vi "机械臂参数配置（数组）.vi"() -> (0 "机械臂臂长":dbl[](array[numeric]), 1 "转轴最大角度":dbl[](array[numeric]), 2 "转轴最小角度":dbl[](array[numeric]))   [LabVIEW 2014]
uses:
  <vilib>/Utility/file.llb/Write To Spreadsheet File (DBL).vi
  <vilib>/Utility/file.llb/Read From Spreadsheet File (DBL).vi
panel:
  in  "取消按钮":bool
  in  "打开配置":bool
  in  "保存配置":bool
  in  "确定":bool
  out "读取机械臂臂长":dbl[](array[numeric])
  out "读取最大角度":dbl[](array[numeric])
  out "读取轴最小角度":dbl[](array[numeric])
  out "读取数据":dbl[][](array[numeric]) caption="所有行" format="%0.3f"
  out "数据":dbl[][](array[numeric])
  out "机械臂臂长2":dbl[](array[numeric])
  out "转轴最大角度2":dbl[](array[numeric])
  out "转轴最小角度2":dbl[](array[numeric])
  in  "Arm-4":dbl
  in  "Arm-3":dbl
  in  "Arm-2":dbl
  in  "Arm-1":dbl
  in  "3-Axi max":dbl
  in  "3-Axi min":dbl
  in  "2-Axi max":dbl
  in  "2-Axi min":dbl
  in  "6-Axi max":dbl
  in  "6-Axi min":dbl
  in  "5-Axi max":dbl
  in  "5-Axi min":dbl
  in  "4-Axi max":dbl
  in  "4-Axi min":dbl
  in  "1-Axi max":dbl
  in  "1-Axi min":dbl
  # "机器臂参数设置"
  # "机械臂臂长（mm）："
  # "机械臂-4"
  # "机械臂-3"
  # "机械臂-2"
  # "机械臂-1"
  # "最大角度（°）："
  # "最小角度（°）："
  # "转轴-3"
  # "转轴-2"
  # "转轴-6"
  # "转轴-5"
  # "转轴-4"
  # "转轴-1"
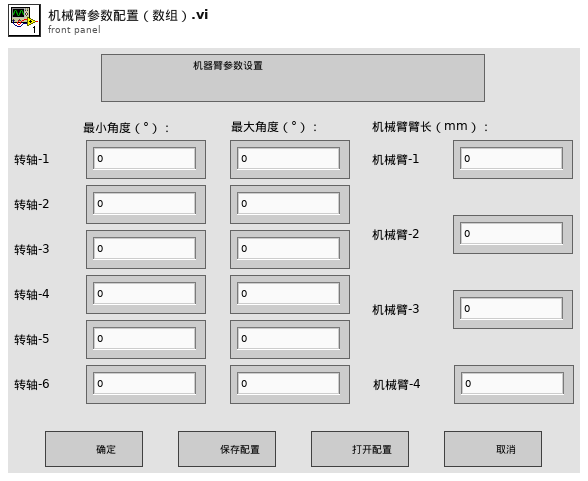
[diagram p1: front panel]
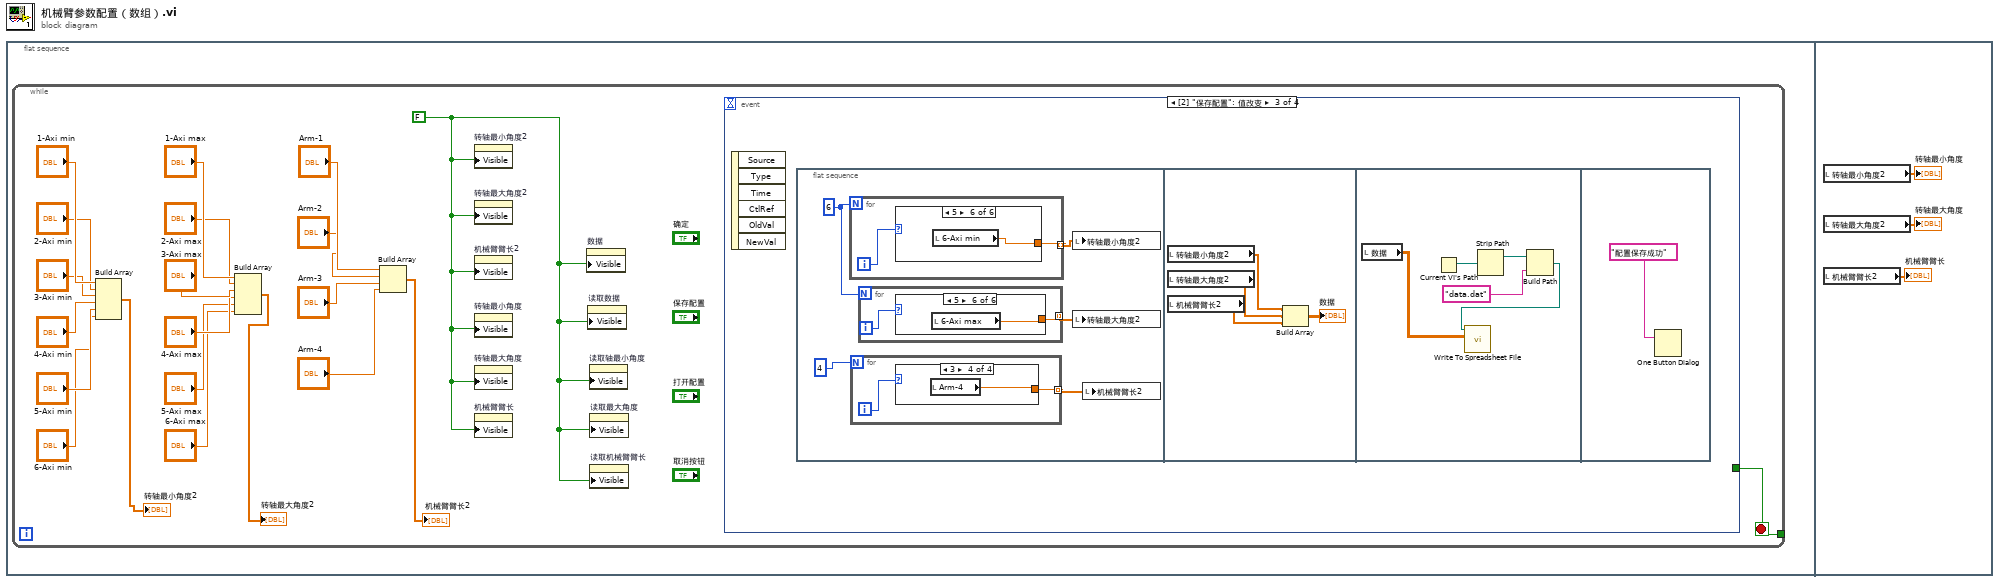
[diagram p0: block diagram]
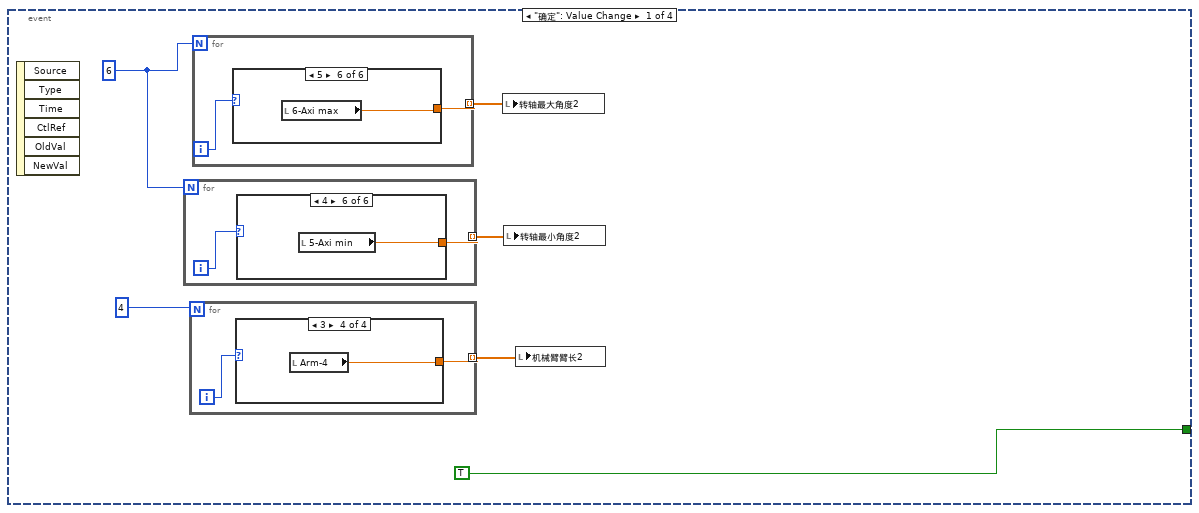
[diagram p2: hidden frame]
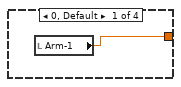
[diagram p3: hidden frame]
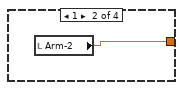
[diagram p4: hidden frame]
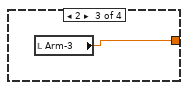
[diagram p5: hidden frame]
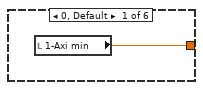
[diagram p6: hidden frame]
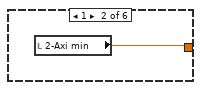
[diagram p7: hidden frame]
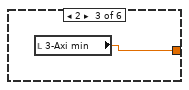
[diagram p8: hidden frame]
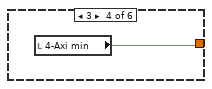
[diagram p9: hidden frame]
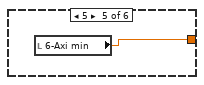
[diagram p10: hidden frame]
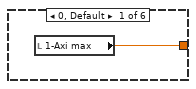
[diagram p11: hidden frame]
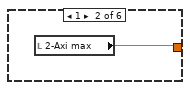
[diagram p12: hidden frame]
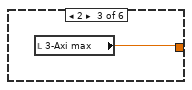
[diagram p13: hidden frame]
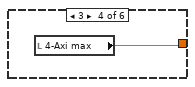
[diagram p14: hidden frame]
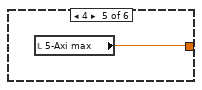
[diagram p15: hidden frame]
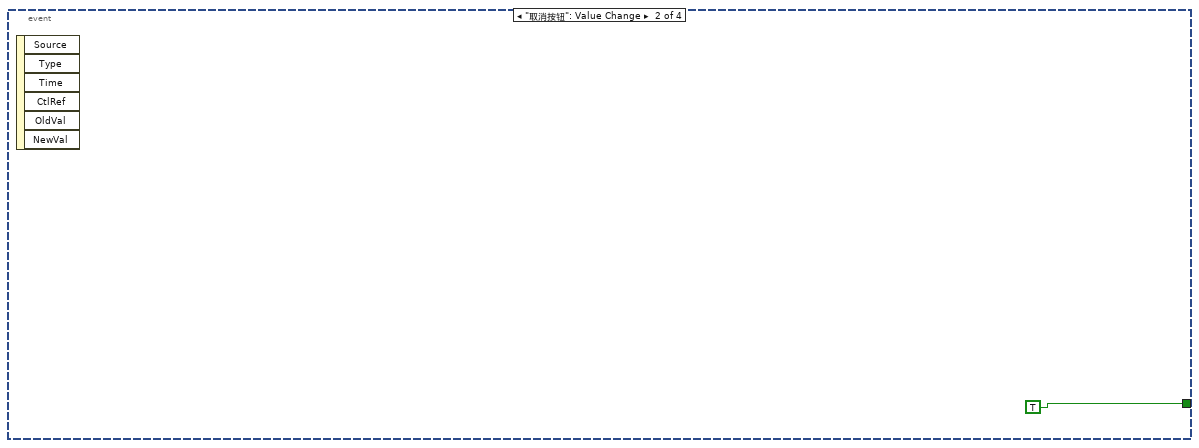
[diagram p16: hidden frame]
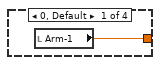
[diagram p17: hidden frame]
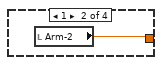
[diagram p18: hidden frame]
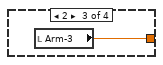
[diagram p19: hidden frame]
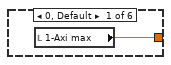
[diagram p20: hidden frame]
diagram:
  n1 = flat-sequence {
    frame #0 {
      n2 = while {
        tunnel: [w5] -> _
        stop <- w5 stop-if-true
        w4 = FALSE
        n3 = Build Array("1-Axi min", "2-Axi min", "3-Axi min", "4-Axi min", "5-Axi min", "6-Axi min") -> (→"转轴最小角度2":dbl[])
        n4 = Build Array("1-Axi max", "2-Axi max", "3-Axi max", "4-Axi max", "5-Axi max", "6-Axi max") -> (→"转轴最大角度2":dbl[])
        n5 = Build Array("Arm-1", "Arm-2", "Arm-3", "Arm-4") -> (→"机械臂臂长2":dbl[])
        n6 = property on="转轴最小角度2" class="Arr (严格)"("Visible"=w4) -> ()  [unwired: 2 in, 2 out]
        n7 = property on="转轴最大角度2" class="Arr (严格)"("Visible"=w4) -> ()  [unwired: 2 in, 2 out]
        n8 = property on="机械臂臂长2" class="Arr (严格)"("Visible"=w4) -> ()  [unwired: 2 in, 2 out]
        n9 = property on="转轴最小角度" class="Arr (严格)"("Visible"=w4) -> ()  [unwired: 2 in, 2 out]
        n10 = property on="转轴最大角度" class="Arr (严格)"("Visible"=w4) -> ()  [unwired: 2 in, 2 out]
        n11 = property on="机械臂臂长" class="Arr (严格)"("Visible"=w4) -> ()  [unwired: 2 in, 2 out]
        n12 = property on="数据" class="Arr (严格)"("Visible"=w4) -> ()  [unwired: 2 in, 2 out]
        n13 = property on="读取数据" class="Arr (严格)"("Visible"=w4) -> ()  [unwired: 2 in, 2 out]
        n14 = property on="读取轴最小角度" class="Arr (严格)"("Visible"=w4) -> ()  [unwired: 2 in, 2 out]
        n15 = property on="读取最大角度" class="Arr (严格)"("Visible"=w4) -> ()  [unwired: 2 in, 2 out]
        n16 = property on="读取机械臂臂长" class="Arr (严格)"("Visible"=w4) -> ()  [unwired: 2 in, 2 out]
        n17 = event shown="[2] \"保存配置\": 值改变" {
          selector: _ -> [_ _ _ _]
          dyn-events: _ -> [_ _ _ _]
          timeout: _ -> [_ _ _ _]
          tunnel: [TRUE TRUE _ _] -> w5
          event "确定": Value Change {
            w25 = 6
            n18 = event-data() -> ()  [unwired: 1 in, 6 out]
            n19 = for {
              N: w25 -> [_]
              tunnel: [w34] -> w24 mode=indexing
              i -> [w35]
              n20 = case shown="4" w35 {
                tunnel: [w36 w37 w38 w39 w40 w41] -> w34
                frame 0, Default {
                  n21 = local read "1-Axi min"() -> (w36:dbl)
                }
                frame 1 {
                  n22 = local read "2-Axi min"() -> (w37:dbl)
                }
                frame 2 {
                  n23 = local read "3-Axi min"() -> (w38:dbl)
                }
                frame 3 {
                  n24 = local read "4-Axi min"() -> (w39:dbl)
                }
                frame 5 {
                  n25 = local read "6-Axi min"() -> (w40:dbl)
                }
                frame 4 {
                  n26 = local read "5-Axi min"() -> (w41:dbl)
                }
              }
            }
            n27 = for {
              N: 4 -> [_]
              tunnel: [w28] -> w22 mode=indexing
              i -> [w29]
              n28 = case shown="3" w29 {
                tunnel: [w30 w31 w32 w33] -> w28
                frame 0, Default {
                  n29 = local read "Arm-1"() -> (w30:dbl)
                }
                frame 1 {
                  n30 = local read "Arm-2"() -> (w31:dbl)
                }
                frame 2 {
                  n31 = local read "Arm-3"() -> (w32:dbl)
                }
                frame 3 {
                  n32 = local read "Arm-4"() -> (w33:dbl)
                }
              }
            }
            n33 = for {
              N: w25 -> [_]
              tunnel: [w42] -> w26 mode=indexing
              i -> [w43]
              n34 = case shown="5" w43 {
                tunnel: [w44 w45 w46 w47 w48 w49] -> w42
                frame 0, Default {
                  n35 = local read "1-Axi max"() -> (w44:dbl)
                }
                frame 1 {
                  n36 = local read "2-Axi max"() -> (w45:dbl)
                }
                frame 2 {
                  n37 = local read "3-Axi max"() -> (w46:dbl)
                }
                frame 3 {
                  n38 = local read "4-Axi max"() -> (w47:dbl)
                }
                frame 4 {
                  n39 = local read "5-Axi max"() -> (w48:dbl)
                }
                frame 5 {
                  n40 = local read "6-Axi max"() -> (w49:dbl)
                }
              }
            }
            n41 = local write "转轴最大角度2"(w26) -> ()
            n42 = local write "转轴最小角度2"(w24) -> ()
            n43 = local write "机械臂臂长2"(w22) -> ()
          }
          event "取消按钮": Value Change {
            n44 = event-data() -> ()  [unwired: 1 in, 6 out]
          }
          event "保存配置": Value Change {
            n45 = event-data() -> ()  [unwired: 1 in, 6 out]
            n46 = flat-sequence {
              frame #0 {
                w55 = 6
                n47 = for {
                  N: w55 -> [_]
                  tunnel: [w70] -> w53 mode=indexing
                  i -> [w71]
                  n48 = case shown="5" w71 {
                    tunnel: [w72 w73 w74 w75 w76 w77] -> w70
                    frame 0, Default {
                      n49 = local read "1-Axi min"() -> (w72:dbl)
                    }
                    frame 1 {
                      n50 = local read "2-Axi min"() -> (w73:dbl)
                    }
                    frame 2 {
                      n51 = local read "3-Axi min"() -> (w74:dbl)
                    }
                    frame 3 {
                      n52 = local read "4-Axi min"() -> (w75:dbl)
                    }
                    frame 4 {
                      n53 = local read "5-Axi min"() -> (w76:dbl)
                    }
                    frame 5 {
                      n54 = local read "6-Axi min"() -> (w77:dbl)
                    }
                  }
                }
                n55 = for {
                  N: 4 -> [_]
                  tunnel: [w56] -> w51 mode=indexing
                  i -> [w57]
                  n56 = case shown="3" w57 {
                    tunnel: [w58 w59 w60 w61] -> w56
                    frame 0, Default {
                      n57 = local read "Arm-1"() -> (w58:dbl)
                    }
                    frame 1 {
                      n58 = local read "Arm-2"() -> (w59:dbl)
                    }
                    frame 2 {
                      n59 = local read "Arm-3"() -> (w60:dbl)
                    }
                    frame 3 {
                      n60 = local read "Arm-4"() -> (w61:dbl)
                    }
                  }
                }
                n61 = for {
                  N: w55 -> [_]
                  tunnel: [w62] -> w52 mode=indexing
                  i -> [w63]
                  n62 = case shown="5" w63 {
                    tunnel: [w64 w65 w66 w67 w68 w69] -> w62
                    frame 0, Default {
                      n63 = local read "1-Axi max"() -> (w64:dbl)
                    }
                    frame 1 {
                      n64 = local read "2-Axi max"() -> (w65:dbl)
                    }
                    frame 2 {
                      n65 = local read "3-Axi max"() -> (w66:dbl)
                    }
                    frame 3 {
                      n66 = local read "4-Axi max"() -> (w67:dbl)
                    }
                    frame 4 {
                      n67 = local read "5-Axi max"() -> (w68:dbl)
                    }
                    frame 5 {
                      n68 = local read "6-Axi max"() -> (w69:dbl)
                    }
                  }
                }
                n69 = local write "转轴最小角度2"(w53) -> ()
                n70 = local write "转轴最大角度2"(w52) -> ()
                n71 = local write "机械臂臂长2"(w51) -> ()
              }
              frame #1 {
                n72 = local read "转轴最小角度2"() -> (w81:dbl[])
                n73 = local read "转轴最大角度2"() -> (w80:dbl[])
                n74 = local read "机械臂臂长2"() -> (w79:dbl[])
                n75 = Build Array(w81, w80, w79) -> (→"数据":dbl[][])
              }
              frame #2 {
                n76 = local read "数据"() -> (w86:dbl[][])
                n77 = Current VI's Path() -> (path=w85:path)
                n78 = Strip Path(path=w85) -> (stripped path=w84:path)  [unwired: 1 out]
                n79 = Build Path(base path=w84, name or relative path="data.dat") -> (appended path=w82:path)
                n80 = call-poly <vilib>:"Write To Spreadsheet File.vi"("2D data"=w86, "file path (dialog if empty)"=w82) -> ()  [unwired: 6 in, 1 out]
              }
              frame #3 {
                n81 = One Button Dialog(message="配置保存成功") -> ()  [unwired: 1 in, 1 out]
              }
            }
          }
          event "打开配置": Value Change {
            n82 = event-data() -> ()  [unwired: 1 in, 6 out]
            n83 = flat-sequence {
              frame #0 {
                n84 = call-poly <vilib>:"Read From Spreadsheet File.vi"() -> ("all rows"=→"读取数据":dbl[][])  [unwired: 7 in, 4 out]
              }
              frame #1 {
                n85 = for {
                  N: 3 -> [_]
                  i -> [w90]
                  n86 = local read "读取数据"() -> (w92:dbl[][])
                  n87 = Index Array(array=w92, index (row)=w90) -> (element=w91:dbl[])  [unwired: 1 in]
                  n88 = case shown="0, 默认" w90 {
                    tunnel: w91 -> [w93 w94 w95]
                    frame 0, Default {
                      "读取轴最小角度" <- w93
                    }
                    frame 1 {
                      "读取最大角度" <- w94
                    }
                    frame 2 {
                      "读取机械臂臂长" <- w95
                    }
                  }
                }
              }
              frame #2 {
                w97 = 6
                n89 = for {
                  N: 4 -> [_]
                  i -> [w98]
                  n90 = local read "读取机械臂臂长"() -> (w100:dbl[])
                  n91 = Index Array(array=w100, index=w98) -> (element=w99:dbl)
                  n92 = case shown="3" w98 {
                    tunnel: w99 -> [w101 w102 w103 w104]
                    frame 0, Default {
                      n93 = local write "Arm-1"(w101) -> ()
                    }
                    frame 1 {
                      n94 = local write "Arm-2"(w102) -> ()
                    }
                    frame 2 {
                      n95 = local write "Arm-3"(w103) -> ()
                    }
                    frame 3 {
                      n96 = local write "Arm-4"(w104) -> ()
                    }
                  }
                }
                n97 = for {
                  N: w97 -> [_]
                  i -> [w105]
                  n98 = local read "读取最大角度"() -> (w107:dbl[])
                  n99 = Index Array(array=w107, index=w105) -> (element=w106:dbl)
                  n100 = case shown="5" w105 {
                    tunnel: w106 -> [w108 w109 w110 w111 w112 w113]
                    frame 0, Default {
                      n101 = local write "1-Axi max"(w108) -> ()
                    }
                    frame 1 {
                      n102 = local write "2-Axi max"(w109) -> ()
                    }
                    frame 2 {
                      n103 = local write "3-Axi max"(w110) -> ()
                    }
                    frame 3 {
                      n104 = local write "4-Axi max"(w111) -> ()
                    }
                    frame 4 {
                      n105 = local write "5-Axi max"(w112) -> ()
                    }
                    frame 5 {
                      n106 = local write "6-Axi max"(w113) -> ()
                    }
                  }
                }
                n107 = for {
                  N: w97 -> [_]
                  i -> [w114]
                  n108 = local read "读取轴最小角度"() -> (w116:dbl[])
                  n109 = Index Array(array=w116, index=w114) -> (element=w115:dbl)
                  n110 = case shown="0, 默认" w114 {
                    tunnel: w115 -> [w117 w118 w119 w120 w121 w122]
                    frame 0, Default {
                      n111 = local write "1-Axi min"(w117) -> ()
                    }
                    frame 1 {
                      n112 = local write "2-Axi min"(w118) -> ()
                    }
                    frame 2 {
                      n113 = local write "3-Axi min"(w119) -> ()
                    }
                    frame 3 {
                      n114 = local write "4-Axi min"(w120) -> ()
                    }
                    frame 4 {
                      n115 = local write "5-Axi min"(w121) -> ()
                    }
                    frame 5 {
                      n116 = local write "6-Axi min"(w122) -> ()
                    }
                  }
                }
              }
            }
          }
        }
      }
    }
    frame #1 {
      n117 = local read "转轴最小角度2"() -> (→"转轴最小角度":dbl[])
      n118 = local read "转轴最大角度2"() -> (→"转轴最大角度":dbl[])
      n119 = local read "机械臂臂长2"() -> (→"机械臂臂长":dbl[])
    }
  }
